vi "Single Shimmer.vi"() -> ()   [LabVIEW 2025]
uses:
  C:/ShimmerLV_Test/ShimmerLVWrapper.dll
  ShimmerLVWrapper.dll
panel:
  out "Waveform Chart":cluster{dbl, dbl, dbl}(graph)
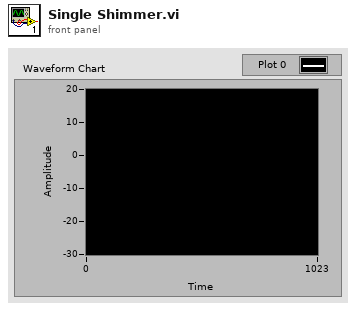
[diagram p1: front panel]
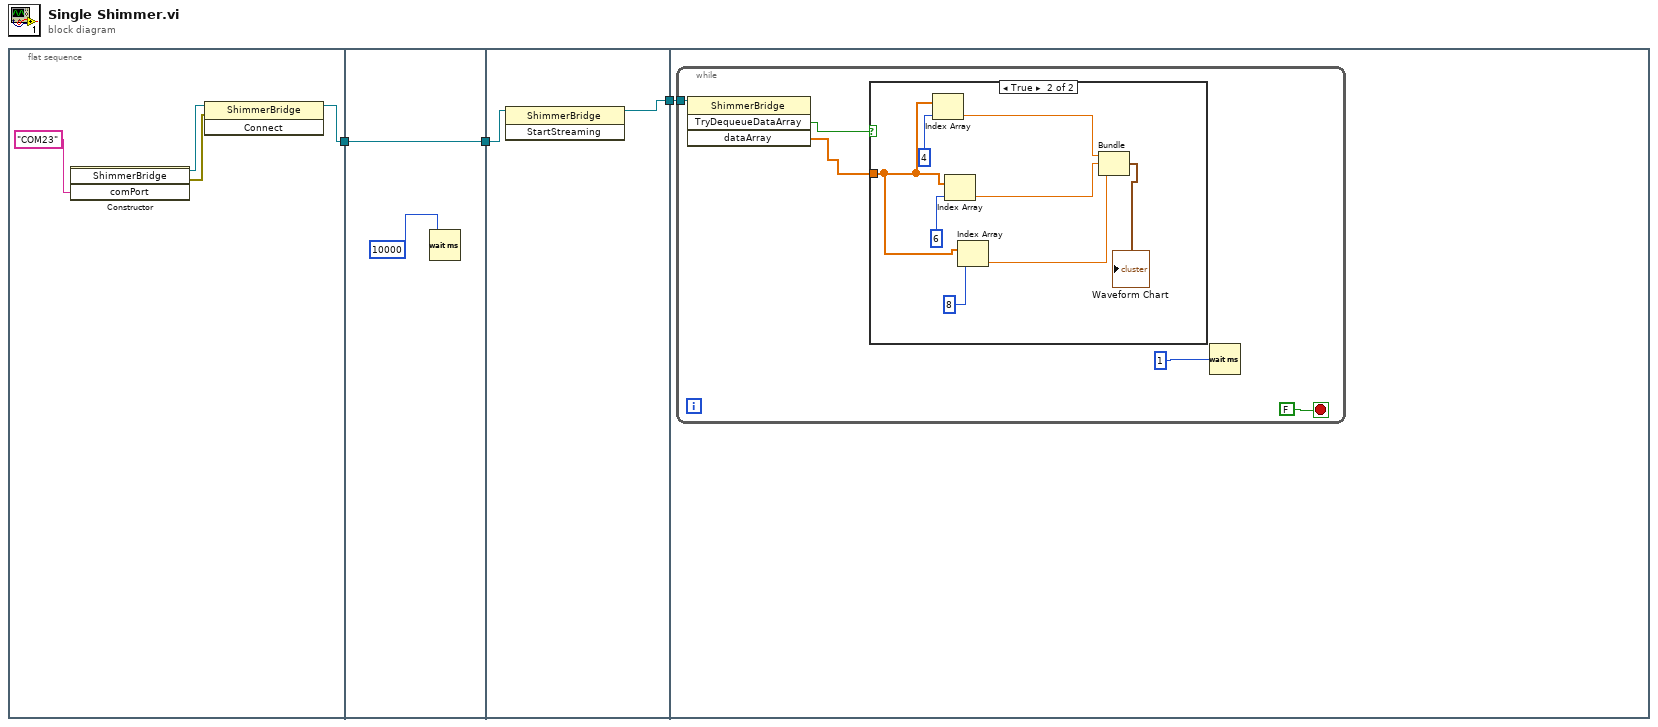
[diagram p0: block diagram]
diagram:
  n1 = flat-sequence {
    tunnel: [w4] -> w3
    tunnel: w3 -> [w8]
    tunnel: [w8] -> w2
    tunnel: w2 -> [w11]
    tunnel: [w10] -> w1
    tunnel: w1 -> [w12]
    frame #0 {
      n2 = constructor class="ShimmerBridge"("comPort"="COM23") -> (reference out=w6:refnum<k24>, error out=w5:errorcluster)  [unwired: 3 in, 2 out]
      n3 = invoke class="ShimmerBridge" method="Connect"(reference=w6, error in=w5) -> (reference out=w4:refnum<k24>)  [unwired: 1 in, 2 out]
    }
    frame #1 {
      n4 = Wait (ms)(milliseconds to wait=u32 10000 ("millisecond timer value")) -> ()  [unwired: 1 out]
    }
    frame #2 {
      n5 = invoke class="ShimmerBridge" method="StartStreaming"(reference=w11) -> (reference out=w10:refnum<k24>)  [unwired: 2 in, 2 out]
    }
    frame #3 {
      n6 = while {
        tunnel: w12 -> [w15]
        stop <- FALSE stop-if-true
        n7 = invoke class="ShimmerBridge" method="TryDequeueDataArray"(reference=w15) -> ("TryDequeueDataArray"=w14:bool, "dataArray"=w13:dbl[])  [unwired: 3 in, 2 out]
        n8 = case shown="True" w14 {
          tunnel: w13 -> [_ w22]
          frame False {
          }
          frame True {
            n9 = Index Array(array=w22, index=4) -> (element=w21:dbl)
            n10 = Index Array(array=w22, index=6) -> (element=w20:dbl)
            n11 = Index Array(array=w22, index=8) -> (element=w19:dbl)
            n12 = Bundle(w21, w20, w19) -> (→"Waveform Chart":cluster{dbl, dbl, dbl})  [unwired: 1 in]
          }
        }
        n13 = Wait (ms)(milliseconds to wait=u32 1) -> ()  [unwired: 1 out]
      }
    }
  }
